vi "Acquisition_numerique.vi"() -> ()   [LabVIEW 2017]
panel:
  out "Pluviometrie":bool caption="données"
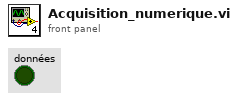
[diagram p1: front panel]
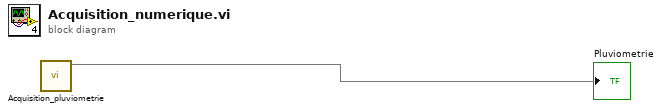
[diagram p0: block diagram]
diagram:
  n1 = call "Acquisition_pluviometrie.vi"() -> (3:→"Pluviometrie")  [unwired: 11 in]
